vi "Array_X_multipleY_worksheet.vi"(0 "Sort?":bool, 1 "column extension":string[](array[string]), 2 "file path (dialog if empty)":path, 3 "Y-column names":string[](array[string]), 5 "graph file":cluster{"all rows":dbl[], "all rows":dbl[]}[](array[cluster]) {"all rows" format="%.2e"; "all rows" format="%.2f"}, 6 "x-column name":string="Xaxis", 7 "export":T1(ring)) -> (4 "Graph array":cluster{"output":dbl[], "output":dbl[]}[](array[cluster]), 8 "new y-column names":string[](array[string]))   [LabVIEW 2019]
uses:
  <vilib>/Utility/file.llb/Write To Spreadsheet File (DBL).vi
panel:
  out "concatenated string":string
  out "appended array":dbl[][](array[numeric])
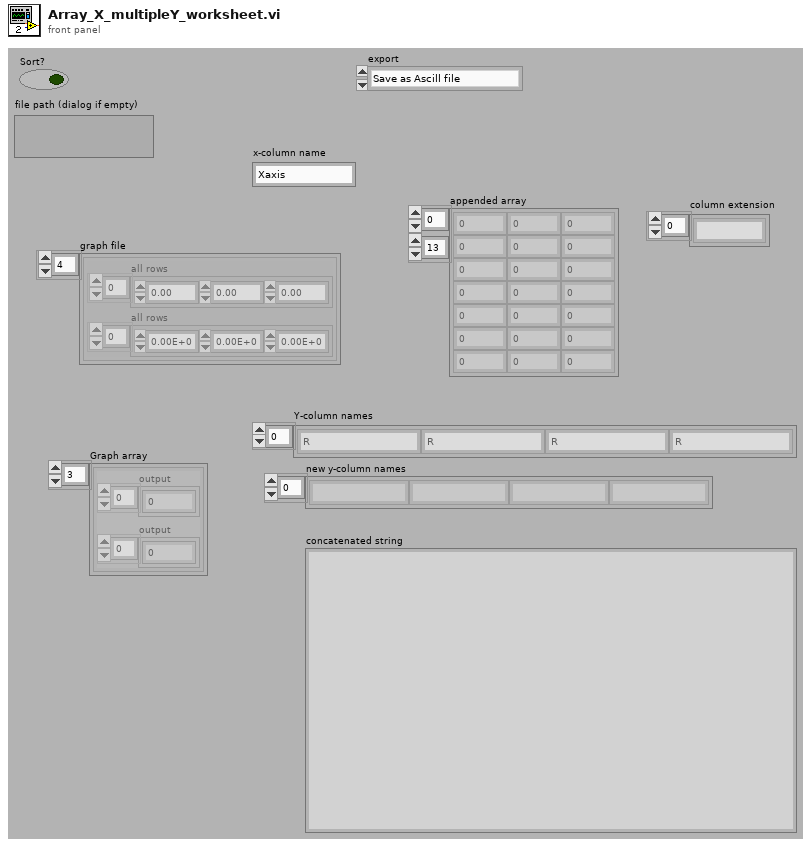
[diagram p1: front panel]
types:
  T1 = enum16{"Save as Ascill file", "write to clipboard", "do not export"}
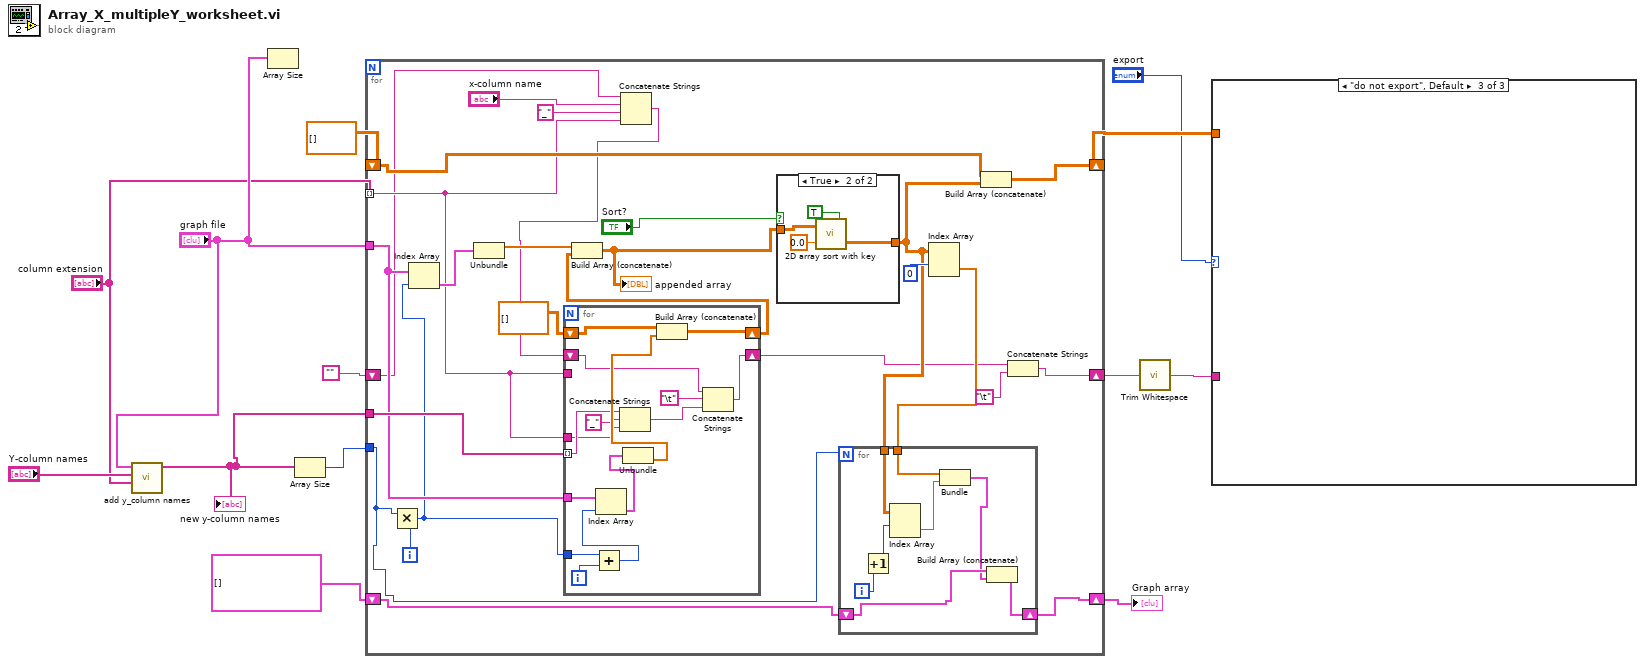
[diagram p0: block diagram]
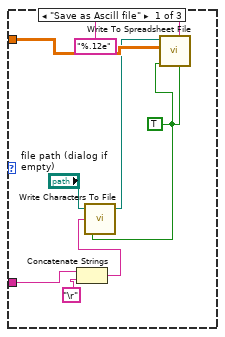
[diagram p2: hidden frame]
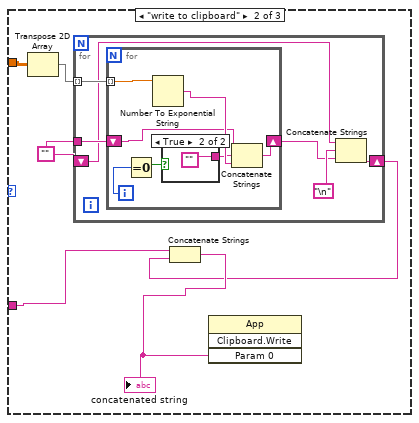
[diagram p3: hidden frame]
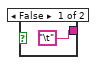
[diagram p4: hidden frame]
diagram:
  n1 = call "add y_column names.vi"("column extension"="column extension", "old y-column names"="Y-column names", "graph file"="graph file") -> ("new y-column names"=w3:string[])  [unwired: 6 in, 2 out]
  "new y-column names" <- w3
  n2 = Array Size(array="graph file") -> ()  [unwired: 1 out]
  n3 = Array Size(array=w3) -> (size(s)=w13:i32)
  n4 = for {
    tunnel: "column extension" -> [w19] mode=indexing
    tunnel: w3 -> [w39]
    tunnel: "graph file" -> [w36]
    tunnel: w13 -> [w29]
    shift-right: [w27] -> w11
    shift-left: cluster{"all rows":sgl[], "all rows":sgl[]}[] [] -> [w28]
    shift-right: [w24] -> w9
    shift-left: dbl[][] [] -> [w22]
    shift-right: [w15] -> w1
    shift-left: "" -> [w17]
    i -> [w37]
    n5 = Multiply(x=w29, y=w37) -> (x*y=w35:i32)
    n6 = Index Array(array=w36, index=w35) -> (element=w38:cluster{"all rows":dbl[], "all rows":dbl[]})
    n7 = Unbundle(w38) -> ("all rows"=w33:dbl[])  [unwired: 1 out]
    n8 = Concatenate Strings(w17, "x-column name", "_" ("string"), w19) -> (w18:string)
    n9 = for {
      tunnel: w39 -> [w59] mode=indexing
      tunnel: w19 -> [_]
      tunnel: w35 -> [w67]
      tunnel: w36 -> [w64]
      shift-right: [w60] -> w31
      shift-left: dbl[][] [] -> [w62]
      tunnel: w19 -> [w57]
      shift-right: [w53] -> w16
      shift-left: w18 -> [w55]
      i -> [w66]
      n10 = Add(x=w67, y=w66) -> (x+y=w65:i32)
      n11 = Index Array(array=w64, index=w65) -> (element=w63:cluster{"all rows":dbl[], "all rows":dbl[]})
      n12 = Concatenate Strings(w59, "_" ("string"), w57) -> (w56:string)
      n13 = Unbundle(w63) -> ("all rows"=w61:dbl[])  [unwired: 1 out]
      n14 = Build Array (concatenate)(w62, w61) -> (w60:dbl[][])
      n15 = Concatenate Strings(w55, "\t", w56) -> (w53:string)
    }
    n16 = Build Array (concatenate)(w33, w31) -> (w26:dbl[][])
    "appended array" <- w26
    n17 = case shown="True" "Sort?" {
      tunnel: w26 -> [w48 w52]
      tunnel: [w48 w49] -> w23
      frame False {
      }
      frame True {
        n18 = call "2D array sort with key.vi"("ascending"=TRUE, "key row"=0.0, "input"=w52) -> ("output"=w49:dbl[][])
      }
    }
    n19 = Index Array(array=w23, index (row)=0 ("disabled index (col)")) -> (element=w30:dbl[])  [unwired: 1 in]
    n20 = for {
      N: w29 -> [_]
      tunnel: w30 -> [w47]
      tunnel: w23 -> [w45]
      shift-right: [w41] -> w27
      shift-left: w28 -> [w43]
      i -> [w46]
      n21 = Increment(x=w46) -> (x+1=w44:i32)
      n22 = Index Array(array=w45, index (row)=w44) -> (element=w40:dbl[])  [unwired: 1 in]
      n23 = Bundle("output"=w47, "output"=w40) -> (w42:cluster{"output":dbl[], "output":dbl[]})  [unwired: 1 out]
      n24 = Build Array (concatenate)(w43, w42) -> (w41:cluster{"output":dbl[], "output":dbl[]}[])
    }
    n25 = Build Array (concatenate)(w22, w23) -> (w24:dbl[][])
    n26 = Concatenate Strings(w16, "\t") -> (w15:string)
  }
  "Graph array" <- w11
  n27 = call <vilib>:"Trim Whitespace.vi"("string"=w1) -> ("trimmed string"=w2:string)  [unwired: 1 in]
  n28 = case shown="\"do not export\", Default" "export" {
    tunnel: w9 -> [w74 w79 _]
    tunnel: w2 -> [w72 w81 _]
    frame "Save as Ascill file" {
      w69 = TRUE
      n29 = Concatenate Strings(w72, "\r") -> (w70:string)
      n30 = call <vilib>:"Write Characters To File.vi"("append to file? (new file:F)"=w69, "character string"=w70, "file path (dialog if empty)"="file path (dialog if empty)") -> ("new file path (Not A Path if cancelled)"=w73:path)  [unwired: 2 out]
      n31 = call-poly <vilib>:"Write To Spreadsheet File.vi"("transpose? (no:F)"=w69, "format (%.3f)"="%.12e", "append to file? (new file:F)"=w69, "2D data"=w74, "file path (dialog if empty)"=w73) -> ()  [unwired: 1 in, 3 out]
    }
    frame "write to clipboard" {
      w77 = ""
      n32 = Transpose 2D Array(2D array=w79) -> (transposed array=w78:dbl[][])
      n33 = for {
        tunnel: w78 -> [w87] mode=indexing
        shift-right: [w86] -> w76
        shift-left: w77 -> [w82]
        tunnel: w77 -> [w85]
        n34 = for {
          tunnel: w87 -> [w94] mode=indexing
          shift-right: [w88] -> w83
          shift-left: w85 -> [w91]
          i -> [w93]
          n35 = Equal To 0?(x=w93) -> (x = 0?=w89:bool)
          n36 = Number To Exponential String(number=w94) -> (E-format string=w92:string)  [unwired: 3 in]
          n37 = case shown="True" w89 {
            tunnel: ["\t" ""] -> w90
            frame False {
            }
            frame True {
            }
          }
          n38 = Concatenate Strings(w91, w90, w92) -> (w88:string)
        }
        n39 = Concatenate Strings(w82, "\n", w83) -> (w86:string)
      }
      n40 = Concatenate Strings(w81, w76) -> (w80:string)
      "concatenated string" <- w80
      n41 = invoke class="App" method="Clipboard.Write"("Param 0"=w80) -> ()  [unwired: 3 in, 4 out]
    }
    frame "do not export", Default {
    }
  }
